vi "Pre Launch Init.vi"(11 "HIJ Vision Launcher in":refnum<class "HIJ Vision Launcher.lvclass">) -> (0 "error out":errorcluster, 3 "HIJ Vision Launcher out":refnum<class "HIJ Vision Launcher.lvclass">)   [LabVIEW 2014, in "HIJ Vision Launcher.lvlib" / "HIJ Vision Launcher.lvclass"]
doc: "(<B>Filename</B>: Actor Framework.lvlib:Actor.lvclass:Pre Launch Init.vi)\n\nDefines behavior that occurs after the Launch Actor method is invoked but before the actor's Actor Core method begins running.\n\nThe Pre Launch Init method is guaranteed to finish before the Launch Actor method returns to its caller and before the actor itself receives any messages. Any references that the Pre Launch Init method obtains are guaranteed to have the same lifetime as the actor itself. Any errors that the Pre Launch Init method returns will abort the launch.\n\nBy default, this method does nothing. A descendant class may override it to define behavior."
uses:
  HIJ Vision Launcher.lvclass
  HIJ Vision Launcher.lvclass/HIJ Vision Launcher.ctl
  Viewable Actor/ViewableActor/ViewableActor.lvclass/ViewableActor.ctl
  Viewable Actor/ViewableActor/Write Config URL.vi
  Viewable Actor/ViewableActorEncaps/ViewableActorEncaps.lvclass
panel:
  out "path":path
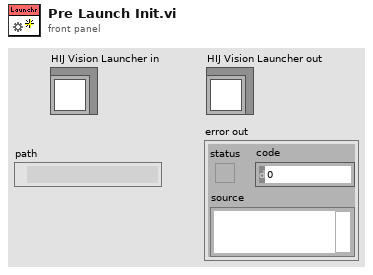
[diagram p1: front panel]
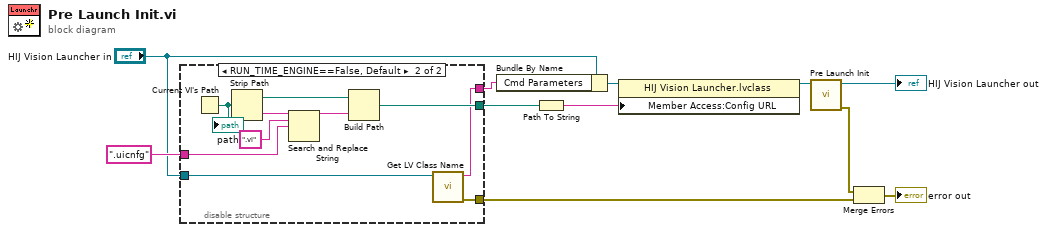
[diagram p0: block diagram]
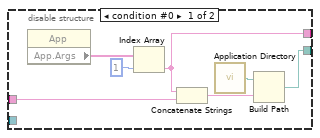
[diagram p2: hidden frame]
diagram:
  n1 = disable-structure shown="RUN_TIME_ENGINE==False, Default" {
    disable-tunnel: [w14 w22] -> w5
    disable-tunnel: ".uicnfg" ("string") -> [w13 w25]
    disable-tunnel: [w12 w20] -> w7
    disable-tunnel: "HIJ Vision Launcher in" -> [_ w21]
    disable-tunnel: [_ w19] -> w1
    frame condition #0 {
      n2 = property class="App"() -> ("App.Args"=w18:string[])  [unwired: 2 in, 2 out]
      n3 = Index Array(array=w18, index=1) -> (element=w12:string)
      n4 = Concatenate Strings(w12, w13) -> (w15:string)
      n5 = call <vilib>:"Application Directory.vi"() -> ("Application Directory"=w16:path)
      n6 = Build Path(base path=w16, name or relative path=w15) -> (appended path=w14:path)
    }
    frame condition #1 (active) {
      n7 = Current VI's Path() -> (path=w28:path)
      "path" <- w28
      n8 = Strip Path(path=w28) -> (stripped path=w23:path, name=w27:string)
      n9 = Search and Replace String(input string=w27, search string=".vi", replace string=w25) -> (result string=w24:string)  [unwired: 5 in, 3 out]
      n10 = Build Path(base path=w23, name or relative path=w24) -> (appended path=w22:path)
      n11 = call <vilib>:"Get LV Class Name.vi"("object"=w21) -> ("error out"=w19:errorcluster, "class name"=w20:string)  [unwired: 9 in]
    }
  }
  n12 = Bundle By Name(cluster="HIJ Vision Launcher in", "Cmd Parameters"=w7) -> (w8:refnum<class "HIJ Vision Launcher.lvclass">)
  n13 = Path To String(path=w5) -> (string=w4:string)
  n14 = property class="HIJ Vision Launcher.lvclass"(reference=w8, "Member Access:Config URL"=w4) -> (reference out=w6:refnum<class "HIJ Vision Launcher.lvclass">)  [unwired: 1 in, 1 out]
  n15 = call-parent "Pre Launch Init.vi"("ViewableActor in"=w6) -> ("error out"=w11:errorcluster, "ViewableActor out"=→"HIJ Vision Launcher out":refnum<class "HIJ Vision Launcher.lvclass">)  [unwired: 9 in]
  n16 = Merge Errors(w11, w1) -> (→"error out":errorcluster)
